vi "GlyphFactory_GetInstance.vi"(8 "error in (no error)":errorcluster, 11 "reference in":refnum<class "GlyphFactory.lvclass"> caption="This control should only be used when\na sub class is inheriting this class") -> (0 "error out":errorcluster, 1 "DVRRefOut":refnum<data-value>, 2 "NewObjectCreated":bool, 3 "reference out":refnum<class "GlyphFactory.lvclass">)   [LabVIEW 2012, in "GlyphFactory.lvclass"]
uses:
  GlyphFactory.lvclass
  ObjectAttributes.ctl
  Character_class/Character.lvclass
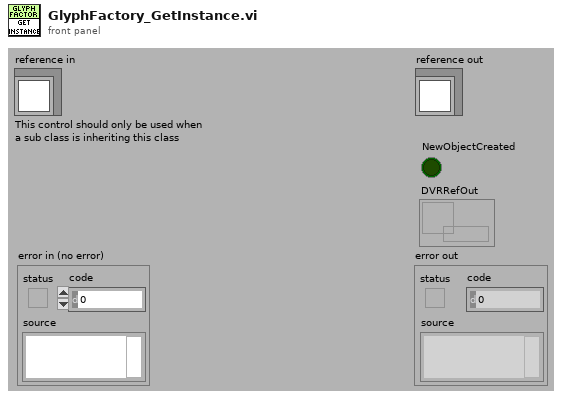
[diagram p1: front panel]
types:
  T1 = enum16{"Create or look up existing", "Look up existing"}
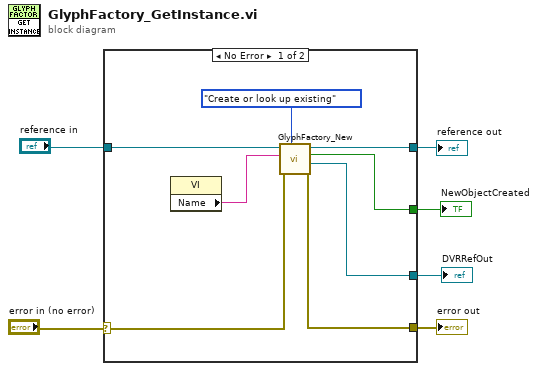
[diagram p0: block diagram]
diagram:
  n1 = case shown="No Error" "error in (no error)" {
    selector: "error in (no error)" -> [w13 w16]
    tunnel: [w14 w15] -> w6
    tunnel: [w12 w16] -> w4
    tunnel: "reference in" -> [w10 w15]
    tunnel: [w9 _] -> w2
    tunnel: [w8 _] -> w1
    frame No Error {
      n2 = property class="VI"() -> ("Name"=w11:string)  [unwired: 2 in, 2 out]
      n3 = call "GlyphFactory_New.vi"("CreateMethod(Create or look up existing)"=T1."Create or look up existing", "error in (no error)"=w13, "Object name"=w11, "reference in"=w10) -> ("error out"=w12:errorcluster, "DVRRefOut"=w8:refnum<data-value>, "NewObjectCreated"=w9:bool, "reference out"=w14:refnum<class "GlyphFactory.lvclass">)  [unwired: 4 in]
    }
    frame Error {
    }
  }
  "reference out" <- w6
  "error out" <- w4
  "NewObjectCreated" <- w2
  "DVRRefOut" <- w1
